vi "_Main_ByRuns_V1.1_3el.vi"() -> ()   [LabVIEW 2017]
uses:
  <vilib>/Instr/_visa.llb/VISA Configure Serial Port (Instr).vi
panel:
  in  "WaveForm":i32(listbox)
  in  "Auto\nturn OFF":bool
  in  "Content":i32(listbox)
  out "LastTrigTimer, s":dbl
  in  "Graph every, cycle":dbl=10.0 min=1.0 max=100.0
  in  "SendPeriod, ms":dbl=100.0 min=10.0 max=10000.0
  out "RunsNeed":i32
  out "DAC1volt, V":dbl
  out "Time LOG":cluster{dbl[], dbl[]}(graph)
  out "LED2":bool
  out "LED1":bool
  out "TrigTimer, s":dbl
  out "Bytes at Port":u32
  out "RecTry":i32
  out "OutVoltage, V":dbl
  out "Field, kV/cm":dbl
  out "VoltageRes, V":dbl
  out "PlotPoints":cluster{"Time":dbl[], "Voltage":dbl[]}(graph)={"Time"=[0.0, 0.00037111111108161925, 0.000510833333311085, 0.0006505555555405509, 0.0007766666666915019, 0.0009172222221968695, 0.0010569444444263353, 0.0011958333333152243, 0.0013350000000274223], "Voltage"=[5.89, 5.89, 5.89, 5.89, 5.89, 5.89, 5.89, 5.89, 5.89]}
  out "VoltageBelow, V":dbl
  in  "Exposition, s":dbl=3.0
  out "Knob":u32
  out "Current, mA":dbl format="%#_4g"
  out "Channel 4, V":dbl format="%#_5g"
  out "Channel 3, V":dbl format="%#_5g"
  out "Channel 2, V":dbl format="%#_5g"
  out "Channel 1, V":dbl format="%#_5g"
  in  "Stop Button":bool
  in  "Start Button":bool
  in  "film H, nm":dbl=50.0
  out "VoltageArray, V":dbl[](array[numeric])
  out "Shutter Red":bool
  out "Shutter Green":bool
  in  "Frames In Run":u32=180
  out "Global Frame Done":u32
  out "Now is Run #":u32
  out "Frame In Run Done":u32
  in  "Step, V":dbl=1.0 min=0.01 max=50.0
  in  "Amplitude, V":dbl=1.0 min=0.1 max=50.0
  in  "LOG file":path
  in  "COM port":refnum<visa-resource-name>
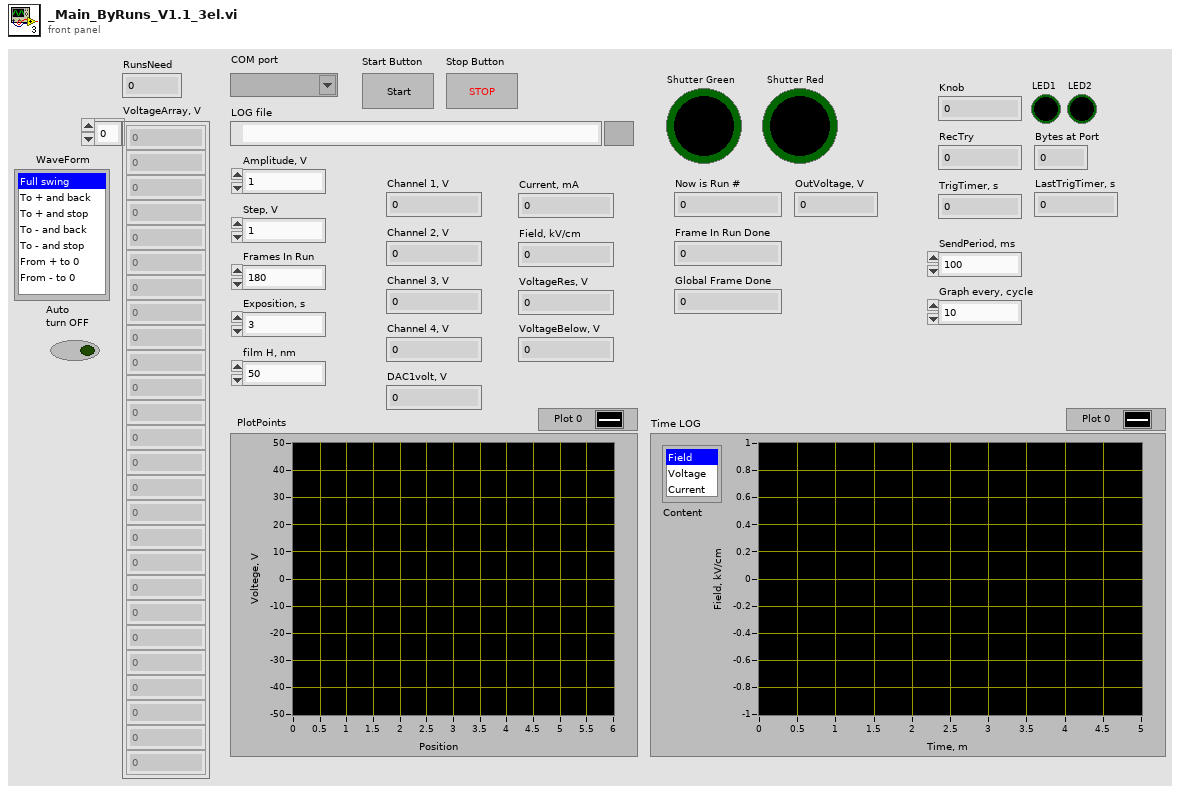
[diagram p1: front panel]
types:
  T1 = cluster{i32, i32, u32, "TrigState":bool, "TrigTimer, s":dbl, "CurrentError":bool}
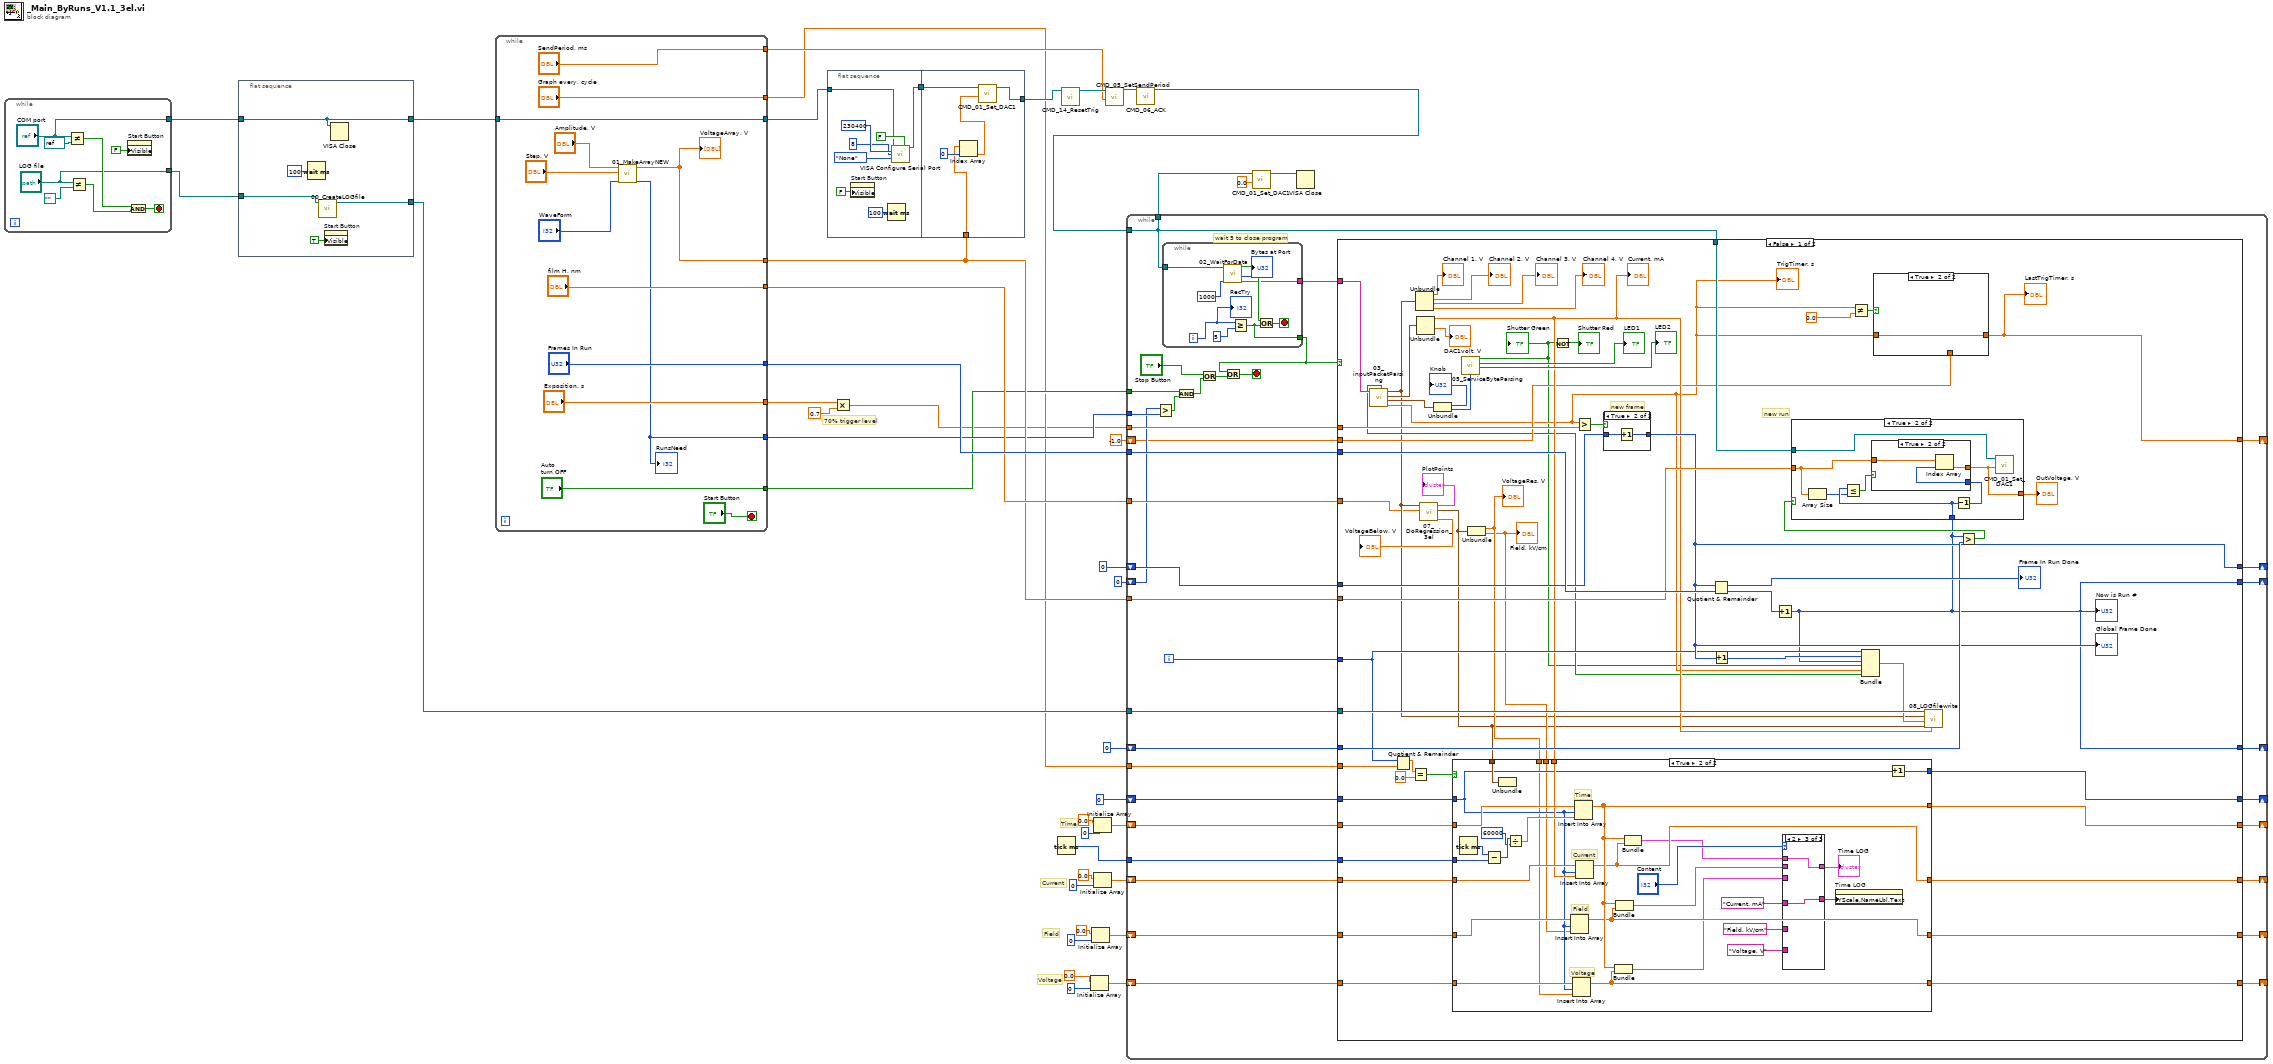
[diagram p0: block diagram]
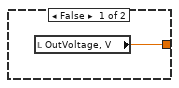
[diagram p6: hidden frame]
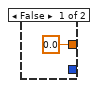
[diagram p7: hidden frame]
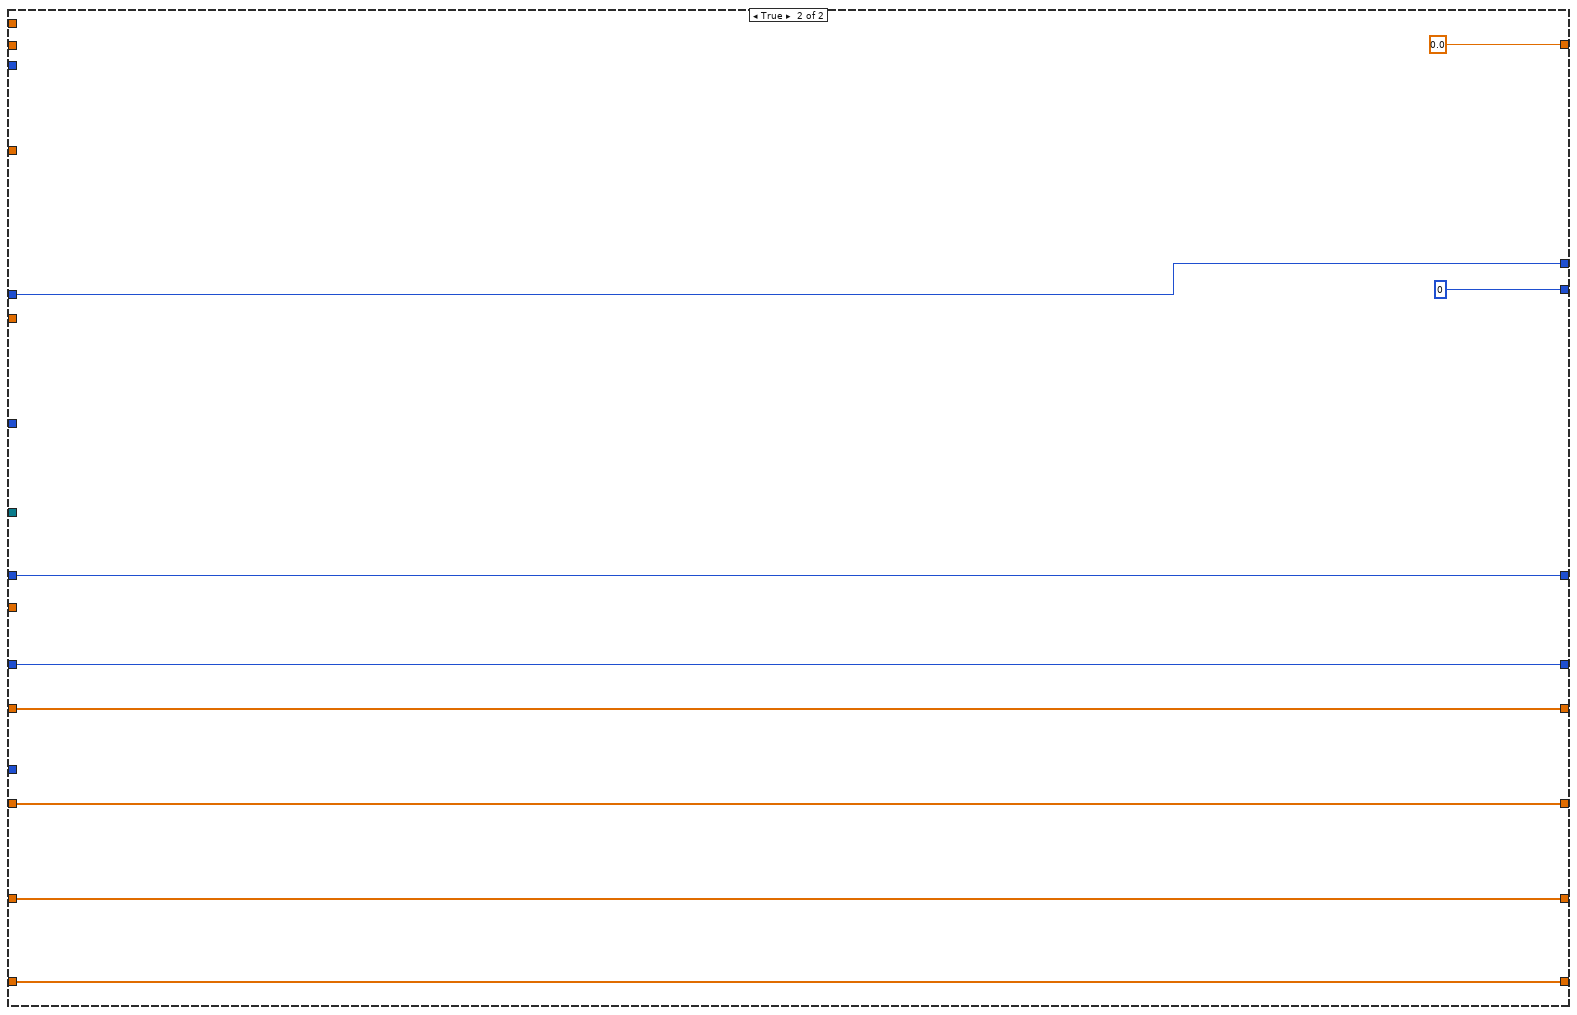
[diagram p9: hidden frame]
diagram:
  # "70% trigger level"
  # "Voltage"
  # "Field"
  # "Time"
  # "Current"
  n1 = while {
    tunnel: ["COM port"] -> w3
    tunnel: ["LOG file"] -> w2
    stop <- w47 stop-if-true
    n2 = Not Equal?(x="COM port", y=refnum<visa-resource-name> refnum ("COM port")) -> (x != y?=w44:bool)
    n3 = Not Equal?(x="LOG file", y=path "" ("LOG file")) -> (x != y?=w45:bool)
    n4 = property on="Start Button" class="Bool"("Visible"=FALSE) -> ()  [unwired: 2 in, 2 out]
    n5 = And(x=w44, y=w45) -> (x .and. y?=w47:bool)
  }
  n6 = flat-sequence {
    tunnel: [w54] -> w38
    tunnel: w3 -> [w50]
    tunnel: w2 -> [w51]
    tunnel: [w50] -> w1
    frame #0 {
      n7 = Wait (ms)(milliseconds to wait=u32 100) -> ()  [unwired: 1 out]
      n8 = call "00_CreateLOGfile.vi"("LOG file"=w51) -> ("refnum out"=w54:refnum<file>)  [unwired: 10 in]
      n9 = property on="Start Button" class="Bool"("Visible"=TRUE) -> ()  [unwired: 2 in, 2 out]
      n10 = VISA Close(VISA resource name=w50) -> ()  [unwired: 1 in, 1 out]
    }
  }
  n11 = while {
    tunnel: w1 -> [w59]
    tunnel: [w59] -> w41
    tunnel: [w56] -> w27
    tunnel: ["film H, nm"] -> w39
    tunnel: ["Frames In Run"] -> w40
    tunnel: ["Exposition, s"] -> w12
    tunnel: [w55] -> w18
    tunnel: ["Auto\nturn OFF"] -> w16
    tunnel: ["SendPeriod, ms"] -> w15
    tunnel: ["Graph every, cycle"] -> w14
    stop <- "Start Button" stop-if-true
    n12 = call "01_MakeArrayNEW.vi"("Amp"="Amplitude, V", "Step"="Step, V", "WaveForm"="WaveForm") -> ("Array"=w56:dbl[], "ArraySize"=w55:i32)  [unwired: 6 in]
    "VoltageArray, V" <- w56
    "RunsNeed" <- w55
  }
  n13 = flat-sequence {
    tunnel: w41 -> [w71]
    tunnel: [w70] -> w28
    tunnel: [w78] -> w34
    tunnel: w28 -> [w77]
    tunnel: w27 -> [w76]
    frame #0 {
      n14 = property on="Start Button" class="Bool"("Visible"=FALSE) -> ()  [unwired: 2 in, 2 out]
      n15 = Wait (ms)(milliseconds to wait=u32 100) -> ()  [unwired: 1 out]
      n16 = call-poly "VISA Configure Serial Port"("VISA resource name"=w71, "Enable Termination\nChar (T)"=FALSE ("Enable Termination\nChar (T)"), "baud rate (9600)"=u32 230400, "data bits (8)"=u16 8, "parity (0:none)"=enum16{"None", "Odd", "Even", "Mark", "Space"}."None") -> ("VISA resource name out"=w70:refnum<visa-resource-name>)  [unwired: 9 in, 1 out]
    }
    frame #1 {
      n17 = Index Array(array=w76, index=0) -> (element=w80:dbl)
      n18 = call "CMD_01_Set_DAC1.vi"("Input, V"=w80, "VISA resource name"=w77) -> ("VISA resource name out"=w78:refnum<visa-resource-name>)  [unwired: 9 in]
    }
  }
  n19 = Multiply(x=w12, y=0.7) -> (x*y=w13:dbl)
  n20 = Tick Count (ms)() -> (millisecond timer value=w22:u32)
  n21 = call "CMD_14_ResetTrig.vi"("VISA resource name"=w34) -> ("VISA resource name out"=w31:refnum<visa-resource-name>)  [unwired: 10 in]
  n22 = Initialize Array(0.0 ("element"), 0 ("dimension size")) -> (w4:dbl[])
  n23 = Initialize Array(0.0 ("element"), 0 ("dimension size")) -> (w5:dbl[])
  n24 = Initialize Array(0.0 ("element"), 0 ("dimension size")) -> (w19:dbl[])
  n25 = Initialize Array(0.0 ("element"), 0 ("dimension size")) -> (w23:dbl[])
  n26 = call "CMD_05_SetSendPeriod.vi"("Period, ms"=w15, "VISA resource name"=w31) -> ("VISA resource name out"=w30:refnum<visa-resource-name>)  [unwired: 9 in]
  n27 = call "CMD_06_ACK.vi"("VISA resource name"=w30) -> ("VISA resource name out"=w29:refnum<visa-resource-name>)  [unwired: 10 in]
  n28 = while {
    tunnel: w29 -> [w103]
    tunnel: [w103] -> w35
    tunnel: w27 -> [w104]
    tunnel: w40 -> [w110]
    tunnel: w13 -> [w112]
    tunnel: w39 -> [w113]
    tunnel: w38 -> [w111]
    shift-right: [w107] -> _
    shift-left: 0 -> [w109]
    shift-right: [w106] -> _
    shift-left: u32 0 -> [w105]
    shift-right: [w101] -> _
    shift-left: 0 -> [w102]
    tunnel: w22 -> [w99]
    shift-right: [w97] -> _
    shift-left: w23 -> [w100]
    shift-right: [w96] -> _
    shift-left: w19 -> [w98]
    tunnel: w18 -> [w92]
    shift-right: [w94] -> _
    shift-left: u32 0 -> [w91]
    tunnel: w16 -> [w88]
    tunnel: w14 -> [w87]
    shift-right: [w86] -> _
    shift-left: -1.0 ("TrigTimer, s") -> [w85]
    shift-right: [w82] -> _
    shift-left: w5 -> [w84]
    shift-right: [w81] -> _
    shift-left: w4 -> [w83]
    i -> [w108]
    stop <- w116 stop-if-true
    # "wait 5 to close program"
    n29 = Greater?(x=w91, y=w92) -> (0:w89:bool)
    n30 = while {
      tunnel: w103 -> [w242]
      tunnel: [w245] -> w115
      tunnel: [w246] -> w114
      i -> [w244]
      stop <- w248 stop-if-true
      n31 = call "02_WaitForData.vi"("WaitTimeoutMS"=u32 1000, "VISA"=w242) -> ("Buffer"=w246:string, "Bytes at Port"=→"Bytes at Port":u32, "Data Recived"=w247:bool)  [unwired: 7 in]
      n32 = Greater Or Equal?(x=w244, y=5) -> (x >= y?=w245:bool)
      n33 = Or(x=w247, y=w245) -> (x .or. y?=w248:bool)
      "RecTry" <- w244
    }
    n34 = And(x=w88, y=w89) -> (x .and. y?=w90:bool)
    n35 = Or(x="Stop Button", y=w90) -> (x .or. y?=w95:bool)
    n36 = Or(x=w115, y=w95) -> (x .or. y?=w116:bool)
    n37 = case shown="False" w115 {
      tunnel: w114 -> [w176 _]
      tunnel: w113 -> [w117 _]
      tunnel: w112 -> [w165 _]
      tunnel: w111 -> [w168 _]
      tunnel: w110 -> [w166 _]
      tunnel: w109 -> [w163 w241]
      tunnel: w108 -> [w147 _]
      tunnel: [w154 w241] -> w107
      tunnel: [w137 w240] -> w106
      tunnel: w105 -> [w157 w240]
      tunnel: w104 -> [w159 _]
      tunnel: w103 -> [w158 _]
      tunnel: w102 -> [w145 w239]
      tunnel: [w144 w239] -> w101
      tunnel: w100 -> [w143 w238]
      tunnel: w99 -> [w142 _]
      tunnel: w98 -> [w141 w237]
      tunnel: [w139 w238] -> w97
      tunnel: [w138 w237] -> w96
      tunnel: [w137 u32 0] -> w94
      tunnel: w87 -> [w135 _]
      tunnel: [w132 0.0 ("TrigTimer, s")] -> w86
      tunnel: w85 -> [w131 _]
      tunnel: w84 -> [w127 w234]
      tunnel: w83 -> [w126 w233]
      tunnel: [w125 w234] -> w82
      tunnel: [w124 w233] -> w81
      frame False {
        # "new run"
        # "new frame"
        n38 = call "03_inputPacketParsing.vi"("string"=w176) -> ("TrigTimer, s"=w130:dbl, "Service state"=w153:cluster{u8, u8}, "DAC state"=w171:cluster{dbl, dbl, dbl, dbl}, "Voltage"=w118:cluster{dbl, dbl, dbl, dbl}, "CurrentError"=w129:bool)  [unwired: 6 in]
        "TrigTimer, s" <- w130
        n39 = Quotient & Remainder(x=w147, y=w135) -> (x-y*floor(x/y)=w149:dbl)  [unwired: 1 out]
        n40 = Equal?(x=w149, y=0.0) -> (x = y?=w146:bool)
        n41 = Unbundle(w118) -> (→"Channel 1, V":dbl, →"Channel 2, V":dbl, →"Channel 3, V":dbl, →"Channel 4, V":dbl)
        n42 = Unbundle(w171) -> (w136:dbl, →"DAC1volt, V":dbl)  [unwired: 2 out]
        "Current, mA" <- w136
        n43 = call "07_DoRegression_3el.vi"("film H, nm"=w117, "Input ChVoltage"=w118) -> ("VoltageBelow, V"=→"VoltageBelow, V":dbl, "Regression"=w120:cluster{"VoltageRes, V":dbl, "Field, kV/cm":dbl}, "PlotPoints"=→"PlotPoints":cluster{"Time":dbl[], "Voltage":dbl[]})  [unwired: 7 in]
        n44 = Unbundle(w153) -> (→"Knob":u8, w152:u8)
        n45 = call "05_ServiceByteParsing.vi"("InputByte"=w152) -> ("LED2"=→"LED2":bool, "LED1"=→"LED1":bool, "TrigState"=w128:bool)  [unwired: 7 in, 1 out]
        "Shutter Green" <- w128
        n46 = Unbundle(w120) -> ("VoltageRes, V"=w123:dbl, "Field, kV/cm"=w122:dbl)
        "VoltageRes, V" <- w123
        "Field, kV/cm" <- w122
        n47 = case shown="True" w146 {
          tunnel: w145 -> [w183 w199]
          tunnel: [w183 w206] -> w144
          tunnel: w120 -> [_ w211]
          tunnel: w143 -> [w181 w204]
          tunnel: w142 -> [_ w209]
          tunnel: w141 -> [w182 w203]
          tunnel: [w182 w193] -> w138
          tunnel: [w181 w196] -> w139
          tunnel: w136 -> [_ w202]
          tunnel: w127 -> [w180 w201]
          tunnel: w126 -> [w179 w200]
          tunnel: [w180 w194] -> w125
          tunnel: [w179 w195] -> w124
          tunnel: w123 -> [_ w197]
          tunnel: w122 -> [_ w198]
          frame False {
          }
          frame True {
            # "Time"
            # "Voltage"
            # "Field"
            # "Current"
            n48 = Tick Count (ms)() -> (millisecond timer value=w210:u32)
            n49 = Subtract(x=w210, y=w209) -> (x-y=w208:u32)
            n50 = Unbundle(w211) -> ()  [unwired: 2 out]
            n51 = Divide(x=w208, y=u32 60000) -> (x/y=w205:dbl)
            n52 = Insert Into Array(array=w201, index=w199, new element=w198) -> (w194:dbl[])
            n53 = Insert Into Array(array=w200, index=w199, new element=w197) -> (w195:dbl[])
            n54 = Insert Into Array(array=w204, index=w199, new element=w205) -> (w196:dbl[])
            n55 = Insert Into Array(array=w203, index=w199, new element=w202) -> (w193:dbl[])
            n56 = Bundle(w196, w195) -> (w189:cluster{dbl[], dbl[]})  [unwired: 1 in]
            n57 = Bundle(w196, w194) -> (w190:cluster{dbl[], dbl[]})  [unwired: 1 in]
            n58 = Bundle(w196, w193) -> (w191:cluster{dbl[], dbl[]})  [unwired: 1 in]
            n59 = case shown="2" "Content" {
              tunnel: w191 -> [_ _ w217]
              tunnel: w190 -> [w213 _ _]
              tunnel: w189 -> [_ w215 _]
              tunnel: [w213 w215 w217] -> w188
              tunnel: "Current, mA" ("Y Scale.Name Label.Text") -> [_ _ w216]
              tunnel: "Field, kV/cm" ("Y Scale.Name Label.Text") -> [w212 _ _]
              tunnel: "Voltage, V" ("Y Scale.Name Label.Text") -> [_ w214 _]
              tunnel: [w212 w214 w216] -> w184
              frame 0, Default {
              }
              frame 1 {
              }
              frame 2 {
              }
            }
            "Time LOG" <- w188
            n60 = property on="Time LOG" class="XYGraph (strict)"("YScale.NameLbl.Text"=w184) -> ()  [unwired: 2 in, 2 out]
            n61 = Increment(x=w199) -> (x+1=w206:i32)
          }
        }
        n62 = Not(x=w128) -> (.not. x?=→"Shutter Red":bool)
        n63 = Greater?(x=w130, y=w165) -> (0:w164:bool)
        n64 = case shown="True" w164 {
          tunnel: w163 -> [w230 w232]
          tunnel: [w230 w231] -> w154
          frame False {
          }
          frame True {
            n65 = Increment(x=w232) -> (x+1=w231:i32)
          }
        }
        "Global Frame Done" <- w154
        n66 = Quotient & Remainder(x=w154, y=w166) -> (x-y*floor(x/y)=→"Frame In Run Done":u32, floor(x/y)=w161:u32)
        n67 = Increment(x=w154) -> (x+1=w155:i32)
        n68 = Increment(x=w161) -> (x+1=w137:u32)
        "Now is Run #" <- w137
        n69 = Not Equal?(x=w130, y=0.0) -> (x != y?=w134:bool)
        n70 = Bundle(w147, w155, w137, "TrigState"=w128, "TrigTimer, s"=w130, "CurrentError"=w129) -> (w167:T1)  [unwired: 1 in]
        n71 = case shown="True" w134 {
          tunnel: [w177 w178] -> w132
          tunnel: w130 -> [_ w178]
          tunnel: w131 -> [w177 _]
          frame False {
          }
          frame True {
          }
        }
        "LastTrigTimer, s" <- w132
        n72 = call "08_LOGfilewrite.vi"("DAC1cur"=w136, "Regression"=w120, "Counters"=w167, "Input ChVoltage"=w118, "refnum out"=w168) -> ()  [unwired: 7 in]
        n73 = Greater?(x=w137, y=w157) -> (0:w162:bool)
        n74 = case shown="True" w162 {
          tunnel: w159 -> [_ w221]
          tunnel: w137 -> [_ w224]
          tunnel: w158 -> [_ w220]
          tunnel: [w218 w219] -> w156
          frame False {
            n75 = local read "OutVoltage, V"() -> (w218:dbl)
          }
          frame True {
            n76 = Array Size(array=w221) -> (size(s)=w223:i32)
            n77 = Less Or Equal?(x=w224, y=w223) -> (x <= y?=w222:bool)
            n78 = Decrement(x=w224) -> (x-1=w225:u32)
            n79 = case shown="True" w222 {
              tunnel: w225 -> [_ w229]
              tunnel: w221 -> [_ w228]
              tunnel: [0.0 w227] -> w219
              frame False {
              }
              frame True {
                n80 = Index Array(array=w228, index=w229) -> (element=w227:dbl)
              }
            }
            n81 = call "CMD_01_Set_DAC1.vi"("Input, V"=w219, "VISA resource name"=w220) -> ()  [unwired: 9 in, 1 out]
          }
        }
        "OutVoltage, V" <- w156
      }
      frame True {
      }
    }
  }
  n82 = call "CMD_01_Set_DAC1.vi"("Input, V"=0.0, "VISA resource name"=w35) -> ("VISA resource name out"=w32:refnum<visa-resource-name>)  [unwired: 9 in]
  n83 = VISA Close(VISA resource name=w32) -> ()  [unwired: 1 in, 1 out]
